vi "Auton-Manipulate.vi"() -> ()   [LabVIEW 2014]
panel:
  in  "Numeric":dbl format="%#_13g"
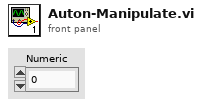
[diagram p1: front panel]
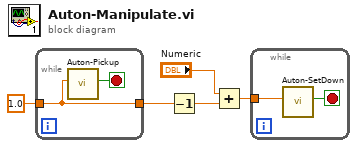
[diagram p0: block diagram]
diagram:
  n1 = while {
    tunnel: [w6] -> w4
    tunnel: 1.0 ("ToHeight") -> [w6]
    stop <- w7 stop-if-true
    n2 = call "Auton-Pickup.vi"("ToHeight"=w6) -> ("Done"=w7:bool)  [unwired: 10 in]
  }
  n3 = Decrement(x=w4) -> (x-1=w1:dbl)
  n4 = Add(x="Numeric", y=w1) -> (x+y=w3:dbl)
  n5 = while {
    tunnel: w3 -> [w8]
    stop <- w9 stop-if-true
    n6 = call "Auton-SetDown.vi"("OnTopOf"=w8) -> ("Boolean"=w9:bool)  [unwired: 10 in]
  }
